vi "WriteCSV.vi"(8 "error in (no error)":errorcluster, 9 "Append file?":bool, 10 "Data to write":string[](array[string]), 11 "CSV file path in":path) -> (0 "error out":errorcluster, 3 "CSV file path out":path)   [LabVIEW 2017, in "LeapMotion.lvlib"]
uses:
  <vilib>/Utility/file.llb/Write Delimited Spreadsheet (string).vi
  LeapMotion.lvlib
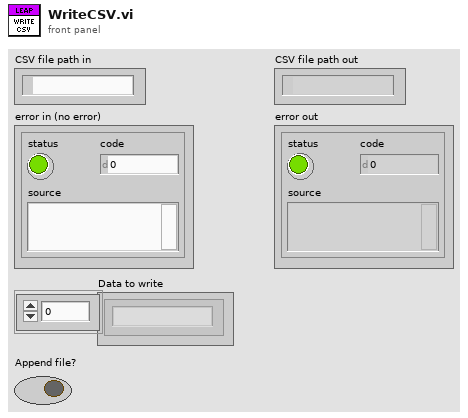
[diagram p1: front panel]
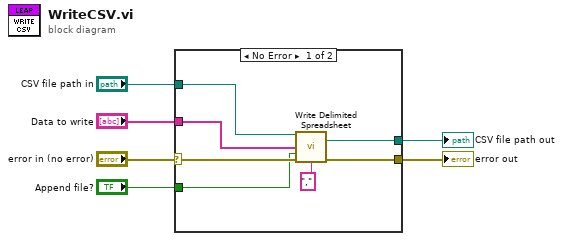
[diagram p0: block diagram]
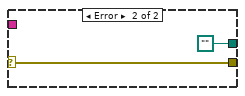
[diagram p2: hidden frame]
diagram:
  n1 = case shown="No Error" "error in (no error)" {
    selector: "error in (no error)" -> [w10 w14]
    tunnel: [w13 w14] -> w6
    tunnel: [w12 path ""] -> w5
    tunnel: "Data to write" -> [w11 _]
    tunnel: "CSV file path in" -> [w9 _]
    tunnel: "Append file?" -> [w7 _]
    frame No Error {
      n2 = call-poly <vilib>:"Write Delimited Spreadsheet.vi"("file path (dialog if empty)"=w9, "1D data"=w11, "append to file? (new file:F)"=w7, "error in (no error)"=w10, "delimiter (\\t)"="," ("delimiter (\\t)")) -> ("new file path (Not A Path if cancelled)"=w12:path, "error out"=w13:errorcluster)  [unwired: 9 in]
    }
    frame Error {
    }
  }
  "error out" <- w6
  "CSV file path out" <- w5
